vi "Aula3-projetoTrifasico.vi"() -> (0 "Tensão Fase B":dynamicdata(graph), 1 "Corrente Fase A":dynamicdata(graph), 2 "Tensão Fase A":dynamicdata(graph), 3 "Corrente Fase B":dynamicdata(graph), 4 "Tensão Fase C":dynamicdata(graph), 5 "Corrente Fase C":dynamicdata(graph), 6 "Timestamp":string[][](table))   [LabVIEW 2025]
panel:
  out "Fase C":string[][](table)
  out "Fase B":string[][](table)
  out "Fase A":string[][](table)
  out "Timestamp":dynamicdata(graph)
  out "All Data":dynamicdata(graph)
  out "All data":string[][](table)
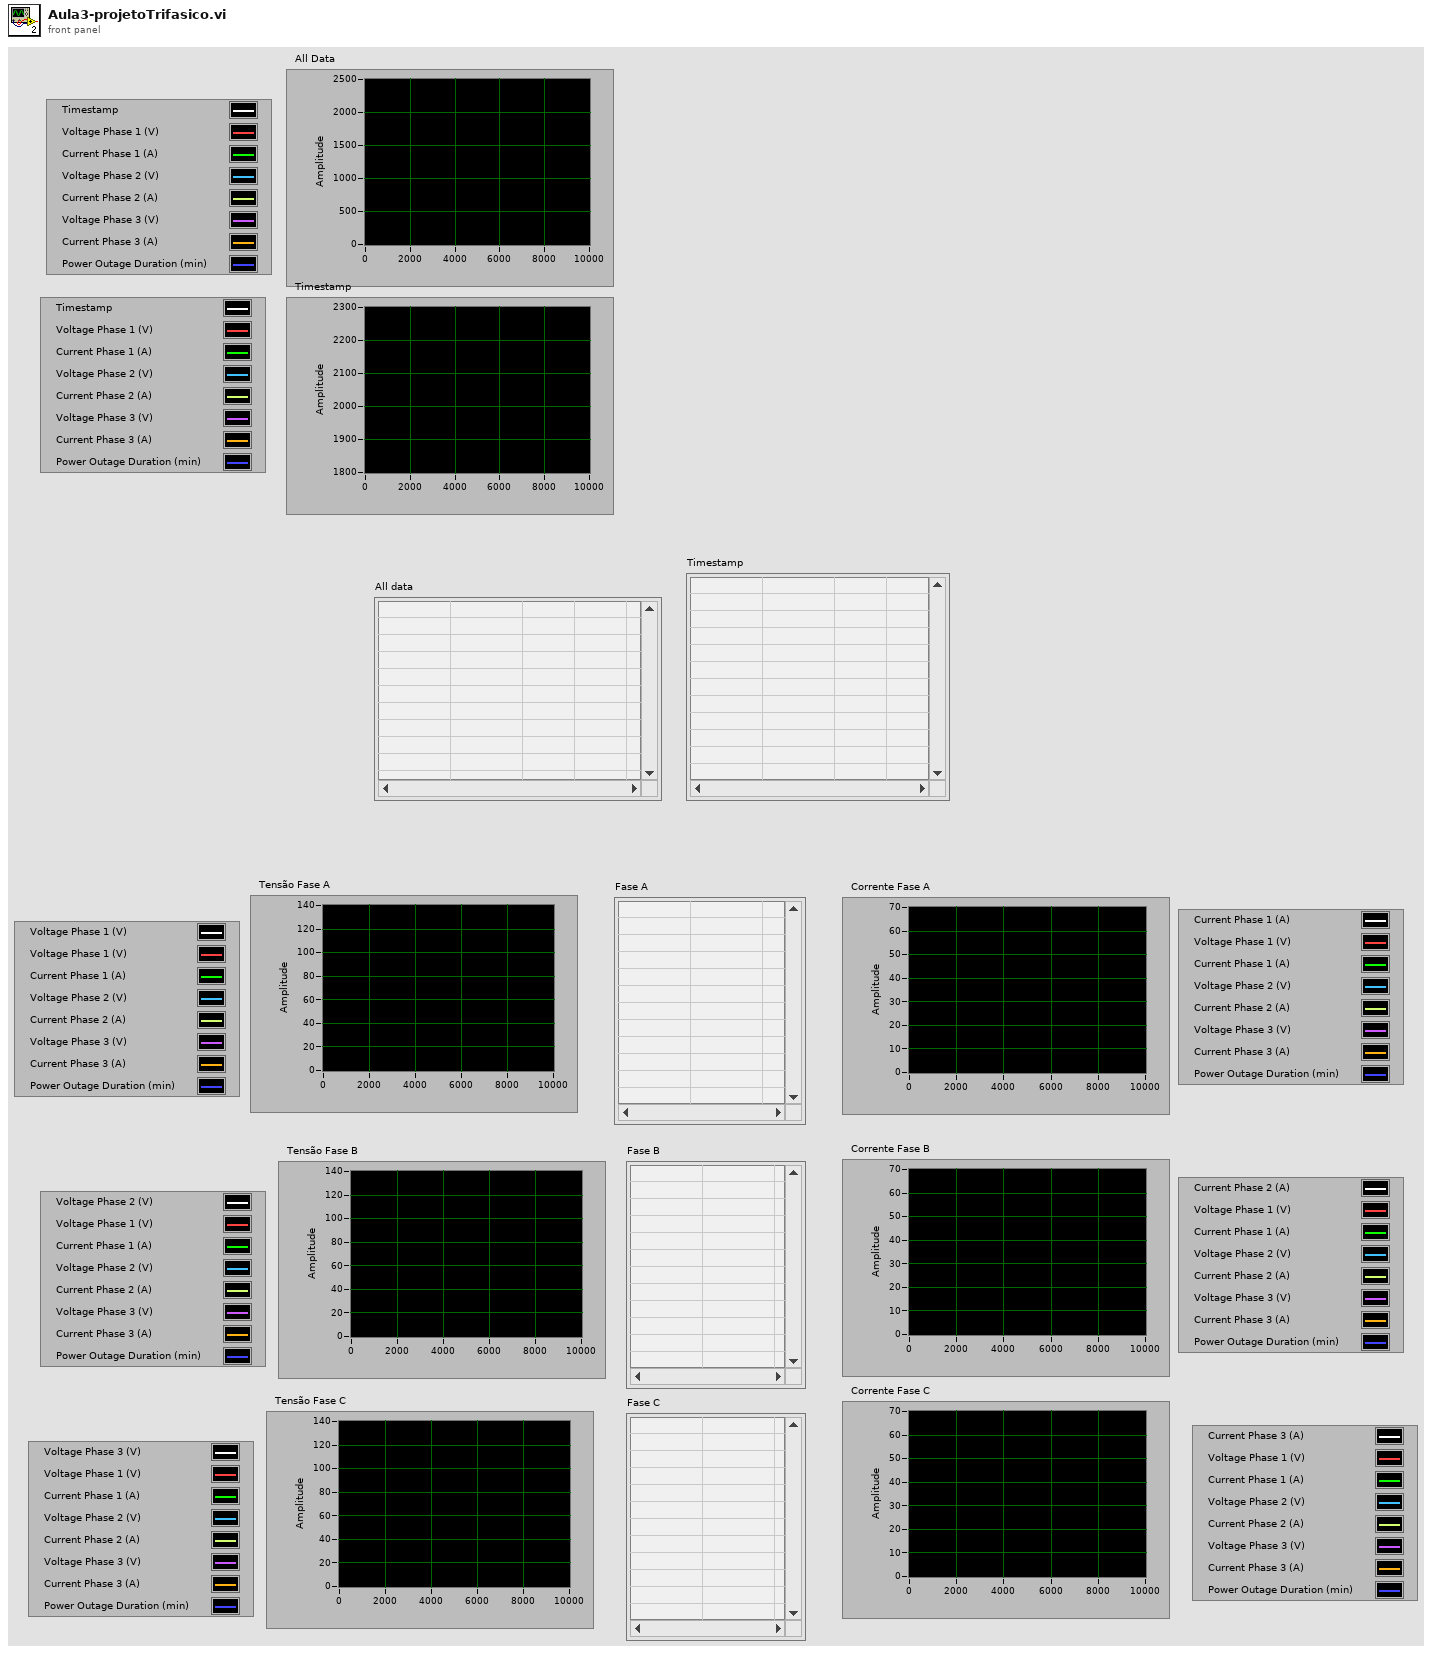
[diagram p1: front panel]
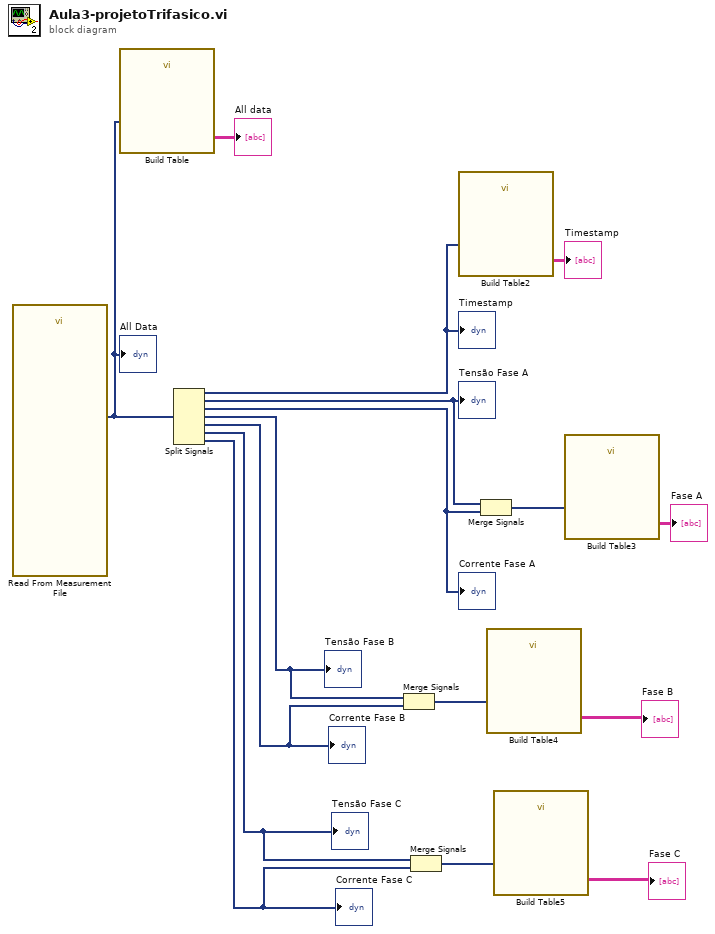
[diagram p0: block diagram]
diagram:
  n1 = call "Read From Measurement File"() -> ("Signals"=w15:dynamicdata)  [unwired: 6 in, 5 out]
  "All Data" <- w15
  n2 = call "Build Table"("Signals"=w15) -> ("Table"=→"All data":string[][])  [unwired: 4 in, 6 out]
  n3 = Split Signals(w15) -> (w13:dynamicdata, w12:dynamicdata, w11:dynamicdata, w8:dynamicdata, w7:dynamicdata, w2:dynamicdata, w1:dynamicdata)  [unwired: 7 in]
  "Timestamp" <- w13
  "Tensão Fase A" <- w12
  "Tensão Fase B" <- w8
  "Corrente Fase B" <- w7
  "Corrente Fase A" <- w11
  "Tensão Fase C" <- w2
  "Corrente Fase C" <- w1
  n4 = Merge Signals(w8, w7) -> (w6:dynamicdata)
  n5 = Merge Signals(w2, w1) -> (w4:dynamicdata)
  n6 = call "Build Table2"("Signals"=w13) -> ("Table"=→"Timestamp":string[][])  [unwired: 4 in, 6 out]
  n7 = Merge Signals(w12, w11) -> (w10:dynamicdata)
  n8 = call "Build Table4"("Signals"=w6) -> ("Table"=→"Fase B":string[][])  [unwired: 4 in, 6 out]
  n9 = call "Build Table5"("Signals"=w4) -> ("Table"=→"Fase C":string[][])  [unwired: 4 in, 6 out]
  n10 = call "Build Table3"("Signals"=w10) -> ("Table"=→"Fase A":string[][])  [unwired: 4 in, 6 out]
